vi "z closure reply.vi"(8 "error in (no error)":errorcluster, 9 "context":u32, 10 "call":u32, 11 "this_":cluster{"_context":u64, "_call":u64}) -> (0 "error out":errorcluster, 1 "context out":u32, 2 "call out":u32, 3 "this_ out":cluster{"_context":u64, "_call":u64})   [LabVIEW 2021, in "zenohc.lvlib"]
doc: "void z_closure_reply(struct z_owned_closure_reply_t *this_,\n void (*call)(struct z_loaned_reply_t *reply, void *context),\n void (*drop)(void *context),\n void *context);"
uses:
  zenohc.lvlib
  zenohc.dll
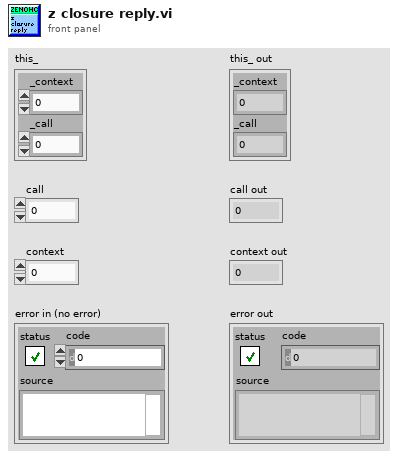
[diagram p1: front panel]
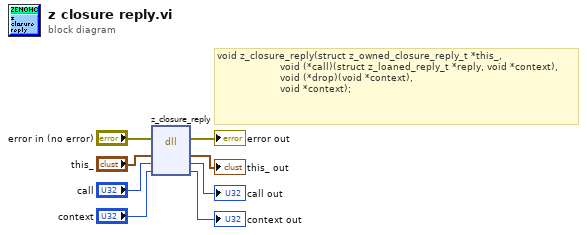
[diagram p0: block diagram]
diagram:
  # "void z_closure_reply(struct z_owned_closure_reply_t *this_,\n                     void (*call)(struct z_loaned_reply_t *reply, void *context),\n                     void (*drop)(void *context),\n                     void *context);"
  n1 = dll-call lib="D:/dev/zenoh_labview/zenohc/zenohc.*" fn="z_closure_reply"(error in="error in (no error)", "this_"="this_", "call"="call", "context"="context") -> (error out=→"error out":errorcluster, "this_"=→"this_ out":cluster{"_context":u64, "_call":u64}, "call"=→"call out":u32, "context"=→"context out":u32)  [unwired: 3 in, 1 out]
